vi "Merge Data.vi"(8 "error in":errorcluster, 10 "Analyzed":refnum<class "Instrument.lvclass">, 11 "Acquired":refnum<class "PAS.lvclass">) -> (0 "error out":errorcluster, 3 "PAS out":refnum<class "PAS.lvclass">)   [LabVIEW 2015, in "PAS Library.lvlib" / "PAS.lvclass"]
doc: "Merge the analyzed data with that of the current retrieved data set. In this case, we are only concerned with insuring that the cell quality and resonant frequency are properly populated."
uses:
  PAS.lvclass
  Instrument/Instrument.lvclass
  Data/Main/PAS Data.lvclass
  Instrument/Instrument.lvclass/Instrument.ctl
  Data/Cell/PAS Cell Data.lvclass/PAS Cell Data.ctl
  Data/Cell/Read IAbackground.vi
  Data/Cell/Write IAbackground.vi
  Instrument/Read Data.vi
  Instrument/Write Data.vi
  Data/Cell/Read derived.vi
  Data/Cell/Write derived.vi
  Data/Data.lvclass
  Data/Cell/PAS Cell Data.lvclass
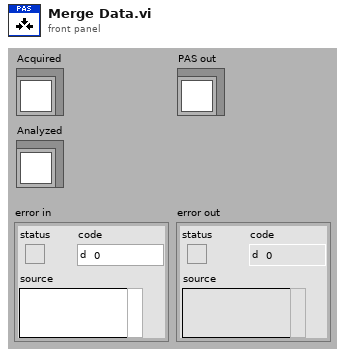
[diagram p1: front panel]
types:
  T1 = cluster{"f0":sgl, "IA":sgl, "Q":sgl, "max":dbl[], "noiseLim":dbl, "ext":dbl}
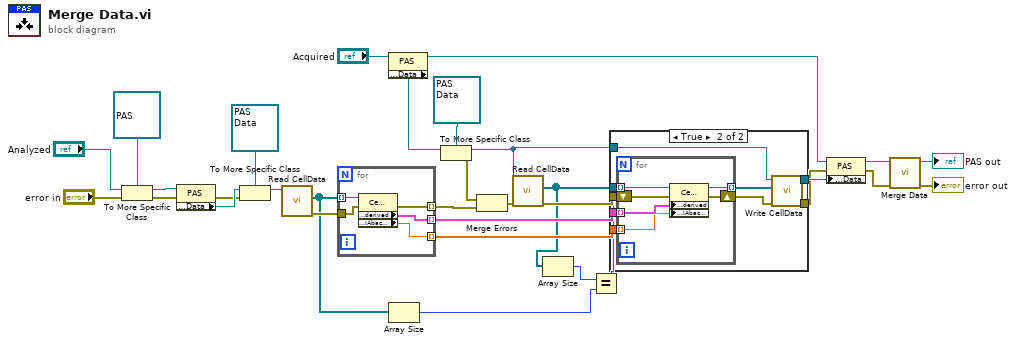
[diagram p0: block diagram]
diagram:
  n1 = To More Specific Class(target class=refnum<class "PAS.lvclass"> refnum ("PAS in"), reference="Analyzed", error in="error in") -> (specific class reference=w13:refnum<class "PAS.lvclass">, error out=w12:errorcluster)
  n2 = property class="PAS"(reference=w13, error in=w12) -> (error out=w11:errorcluster, "Accessors:Data"=w14:refnum<class "Data.lvclass">)  [unwired: 1 out]
  n3 = To More Specific Class(target class=refnum<class "PAS Data.lvclass"> refnum ("Data"), reference=w14, error in=w11) -> (specific class reference=w10:refnum<class "PAS Data.lvclass">)  [unwired: 1 out]
  n4 = call "Read CellData.vi"("PAS Data in"=w10) -> ("error out"=w31:errorcluster, "CellData"=w3:refnum<class "PAS Cell Data.lvclass">[])  [unwired: 8 in, 1 out]
  n5 = for {
    tunnel: w3 -> [w37] mode=indexing
    tunnel: w31 -> [w33]
    tunnel: [w36] -> w30 mode=indexing
    tunnel: [w35] -> w29 mode=indexing
    tunnel: [w34] -> w22 mode=indexing
    n6 = property class="Cell Data"(reference=w37, error in=w33) -> (error out=w35:errorcluster, "Accessors:derived"=w36:T1, "Accessors:IAbackground"=w34:dbl)  [unwired: 1 out]
  }
  n7 = property class="PAS"(reference="Acquired") -> (reference out=w18:refnum<class "PAS.lvclass">, "Accessors:Data"=w21:refnum<class "Data.lvclass">)  [unwired: 1 in, 1 out]
  n8 = Array Size(array=w3) -> (size(s)=w2:i32)
  n9 = To More Specific Class(target class=refnum<class "PAS Data.lvclass"> refnum ("Data"), reference=w21) -> (specific class reference=w19:refnum<class "PAS Data.lvclass">, error out=w8:errorcluster)  [unwired: 1 in]
  n10 = Merge Errors(w8, w29) -> (w23:errorcluster)
  n11 = call "Read CellData.vi"("error in"=w23, "PAS Data in"=w19) -> ("error out"=w32:errorcluster, "CellData"=w5:refnum<class "PAS Cell Data.lvclass">[])  [unwired: 7 in, 1 out]
  n12 = Array Size(array=w5) -> (size(s)=w4:i32)
  n13 = Equal?(x=w4, y=w2) -> (x = y?=w1:bool)
  n14 = case shown="True" w1 {
    tunnel: w32 -> [w38 w47]
    tunnel: w30 -> [_ w45]
    tunnel: w22 -> [_ w44]
    tunnel: w19 -> [w39 w43]
    tunnel: [w39 w42] -> w17
    tunnel: [w38 w41] -> w7
    tunnel: w5 -> [_ w40]
    frame False {
    }
    frame True {
      n15 = for {
        tunnel: w40 -> [w54] mode=indexing
        tunnel: [w51] -> w46 mode=indexing
        tunnel: w45 -> [w50] mode=indexing
        tunnel: w44 -> [w49] mode=indexing
        shift-right: [w52] -> w48
        shift-left: w47 -> [w53]
        n16 = property class="Cell Data"(reference=w54, error in=w53, "Accessors:derived"=w50, "Accessors:IAbackground"=w49) -> (reference out=w51:refnum<class "PAS Cell Data.lvclass">, error out=w52:errorcluster)
      }
      n17 = call "Write CellData.vi"("error in"=w48, "CellData"=w46, "PAS Data in"=w43) -> ("error out"=w41:errorcluster, "PAS Data out"=w42:refnum<class "PAS Data.lvclass">)  [unwired: 7 in]
    }
  }
  n18 = property class="PAS"(reference=w18, error in=w7, "Accessors:Data"=w17) -> (reference out=w15:refnum<class "PAS.lvclass">, error out=w6:errorcluster)
  n19 = call-parent "Merge Data.vi"("error in"=w6, "Acquired"=w15) -> ("error out"=→"error out":errorcluster, "Instrument out"=→"PAS out":refnum<class "PAS.lvclass">)  [unwired: 8 in]
